vi "testLibReader.vi"(8 "error in (no error)":errorcluster) -> (0 "error out":errorcluster)   [LabVIEW 2018]
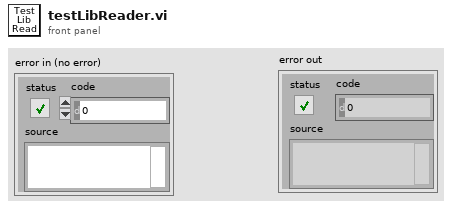
[diagram p1: front panel]
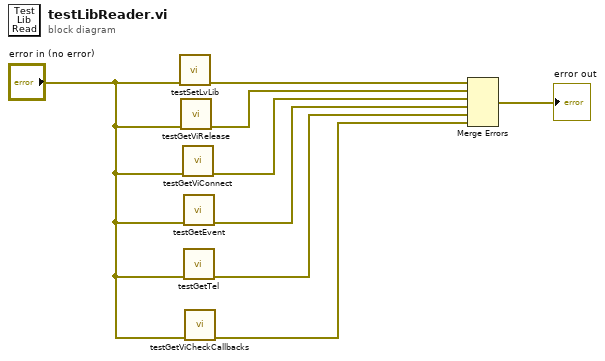
[diagram p0: block diagram]
diagram:
  n1 = call "testSetLvLib.vi"("error in (no error)"="error in (no error)") -> ("error out"=w8:errorcluster)  [unwired: 10 in]
  n2 = call "testGetViRelease.vi"("error in (no error)"="error in (no error)") -> ("error out"=w7:errorcluster)  [unwired: 10 in]
  n3 = call "testGetViConnect.vi"("error in (no error)"="error in (no error)") -> ("error out"=w5:errorcluster)  [unwired: 10 in]
  n4 = call "testGetEvent.vi"("error in (no error)"="error in (no error)") -> ("error out"=w4:errorcluster)  [unwired: 10 in]
  n5 = call "testGetTel.vi"("error in (no error)"="error in (no error)") -> ("error out"=w3:errorcluster)  [unwired: 10 in]
  n6 = call "testGetViCheckCallbacks.vi"("error in (no error)"="error in (no error)") -> ("error out"=w1:errorcluster)  [unwired: 10 in]
  n7 = Merge Errors(w8, w7, w5, w4, w3, w1) -> (→"error out":errorcluster)
